vi "FPGA Server (9636).vi"() -> ()   [LabVIEW 2015]
doc: "This is the FPGA server for the sbRIO for the open-path cavity ring down."
uses:
  Rate.ctl
  <vilib>/Platform/TimedLoop/XDataNode/timing_clust.ctl
  <vilib>/Platform/TimedLoop/XDataNode/nitl_modes.ctl
  <vilib>/Platform/TimedLoop/XDataNode/wakeup.ctl
  <vilib>/rvi/FXPMathLib/FxpDiv/subVIs/nifxpmath_Div_SimConfig.ctl
  <vilib>/rvi/FXPMathLib/basic elements/FxpIntAccumulator/subVIs/nifxpmath_IntAccumulator_SimConfig.ctl
  <vilib>/rvi/Emulation/niFpgaGetClockAttributes.vi
  <vilib>/rvi/Emulation/niFpgaSctlEmulationGetInTimedLoop.vi
  <vilib>/rvi/Emulation/niFpgaEmulationReportErrorSimple.vi
  <vilib>/rvi/Emulation/niFpgaProcessEmulError.vi
  <vilib>/rvi/Memory/Memory_Emulation/nirvimemoryFastEmulation.vi
  <vilib>/rvi/Memory/Memory_Emulation/nirvimemoryEmulation.vi
  <vilib>/rvi/Emulation/niFpgaEmulationIsFPGAContextNoSignature.vi
  <vilib>/rvi/DataTransferAndStorage/Container/Common/niFpgaContainerGetUniqueNameForEmu.vi
  <vilib>/rvi/errors/nirviReportUnexpectedCaseInternalError (U32).vi
  <vilib>/rvi/interface/RandomDataEmulation/niFpgaRandomDataHandleErrors.vi
  <vilib>/rvi/Emulation/niFpgaCriticalErrorInLSC.vi
  <vilib>/rvi/eio/common/nirviEmuTemplateMethod_errors.vi
  <vilib>/rvi/Analysis/common/codeGenErrors/XNode/niFpgaXNodeCodeGenErrorHandle.vi
  <vilib>/rvi/FXPMathLib/basic elements/FxpIntAccumulator/simVIs/DllFxpIntAccumulator_sub.vi
  <vilib>/rvi/FXPMathLib/FxpDiv/simVIs/DllFxpDivTemp_sub.vi
  <vilib>/rvi/DataTransferAndStorage/Container/XNode/niFpgaContainer.xnode
  <vilib>/rvi/interface/RandomDataEmulation/nirviRandomDataFpgaReadWriteTemplate.vi
  <vilib>/eio/EIONode/EIONode.xnode
  <vilib>/rvi/Analysis/measure/mean-var-std/XNode/niFpgaMean-Var-Std.xnode
  <vilib>/Platform/TimedLoop/XDataNode/XDataNode.xnode
  <vilib>/rvi/FXPMathLib/basic elements/FxpIntAccumulator/XNode/nifxpmath_IntAccumulator.xnode
  <vilib>/rvi/FXPMathLib/FxpMul/XNode/nifxpmath_Multiplier.xnode
  <vilib>/rvi/FXPMathLib/FxpSub/XNode/nifxpmath_Sub.xnode
  <vilib>/rvi/FXPMathLib/FxpDiv/XNode/nifxpmath_Div.xnode
  <vilib>/Platform/TimedLoop/XDataNode/XDNodeRunTimeDep.lvlib
  <vilib>/rvi/FXPMathLib/sim/FxpSim.dll
panel:
  out "Rotronic":cluster{"RH":fxp<+,16,8>, "T":fxp<+/-,16,8>}
  out "CollectData":bool
  in  "max":i32
  in  "InvertLaser?":bool
  in  "LaserOff (us)":u32
  in  "Fans":T1
  in  "Reverse?":bool
  out "ShipError":bool
  out "EncodeLoop":bool
  out "ServoLoop":bool
  out "LaserLoop":bool
  out "HKLoop":bool
  out "ShipLoop":bool
  out "DataLoop":bool
  out "LF Data":T2
  in  "Low":u32 caption="Count(uSec)"
  in  "High":u32 caption="Count(uSec)"
  out "Delay Ticks":u32
  in  "Delay (us)":u16
  out "RequestLaser":bool
  out "Sample Ticks":u32
  in  "Pause Digitizer":bool
  in  "Sample Time (us)":u16
  in  "Rate":T3=3 items=["1 MHz"=20, "2 MHz"=10, "2.5 MHz"=8, "5 MHz"=4, "10 MHz"=2, "20MHz"=1]
  out "LaserOFF?":bool
  in  "Cylce (ticks)":u32=40000
  out "DataRead":bool
  out "dataready":bool
  out "NewData":u16
  out "NumElements":u32
  in  "Stop":bool
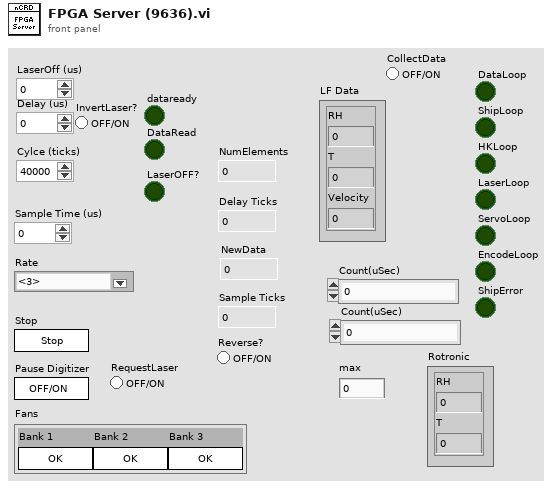
[diagram p1: front panel]
types:
  T1 = cluster{"Bank 1":bool, "Bank 2":bool, "Bank 3":bool}
  T2 = cluster{"RH":fxp<+,16,8>, "T":fxp<+/-,16,8>, "Velocity":fxp<+/-,16,8>}
  T3 = typedef "Rate.ctl" = u8
  T4 = typedef "XDNodeRunTimeDep.lvlib/timing_clust.ctl" = cluster{"Expected End [f-1]":u64, "Actual End [f-1]":u64, "Finished Late? [f-1]":bool, "Expected End [i-1]":u64, "Actual End [i-1]":u64, "Finished Late? [i-1]":bool, "Expected Start [i]":u64, "Actual Start [i]":u64, "Expected Start [f]":u64, "Actual Start [f]":u64, "Source Name":string, "Structure Name":string, "Period":i64, "Deadline":i64, "Offset":i64, "Start":i64, "Priority":i32, "Timeout":i32, "Mode":T5, "Wakeup Reason":T6, "Error":errorcluster, "Source Type":string, "Secondary Source Type":string, "Global End Time":u64, "Global Start Time":u64, "Frame Duration":u64, "Iteration Duration":u64, "Assigned CPU":i32, "I/O Scan Engine Mode":u32}
  T5 = typedef "XDNodeRunTimeDep.lvlib/nitl_modes.ctl" = enum32{"No Change", "Process missed periods, maintain original phase", "Discard missed periods, maintain original phase", "Process missed periods, ignore original phase", "Discard missed periods, ignore original phase"}
  T6 = typedef "XDNodeRunTimeDep.lvlib/wakeup.ctl" = enum32{"Normal", "Aborted", "Asynchronous wakeup", "Timing source error", "Timed loop error", "Timeout"}
  T7 = cluster{"fixed-point type":fxp<+/-,64,64>, "x+y":fxp<+/-,64,64>, "x+y":fxp<+/-,64,64>, "x+y":fxp<+/-,64,64>, "x+y":fxp<+/-,64,64>, "x+y":fxp<+/-,64,64>, "x+y":fxp<+/-,64,64>}
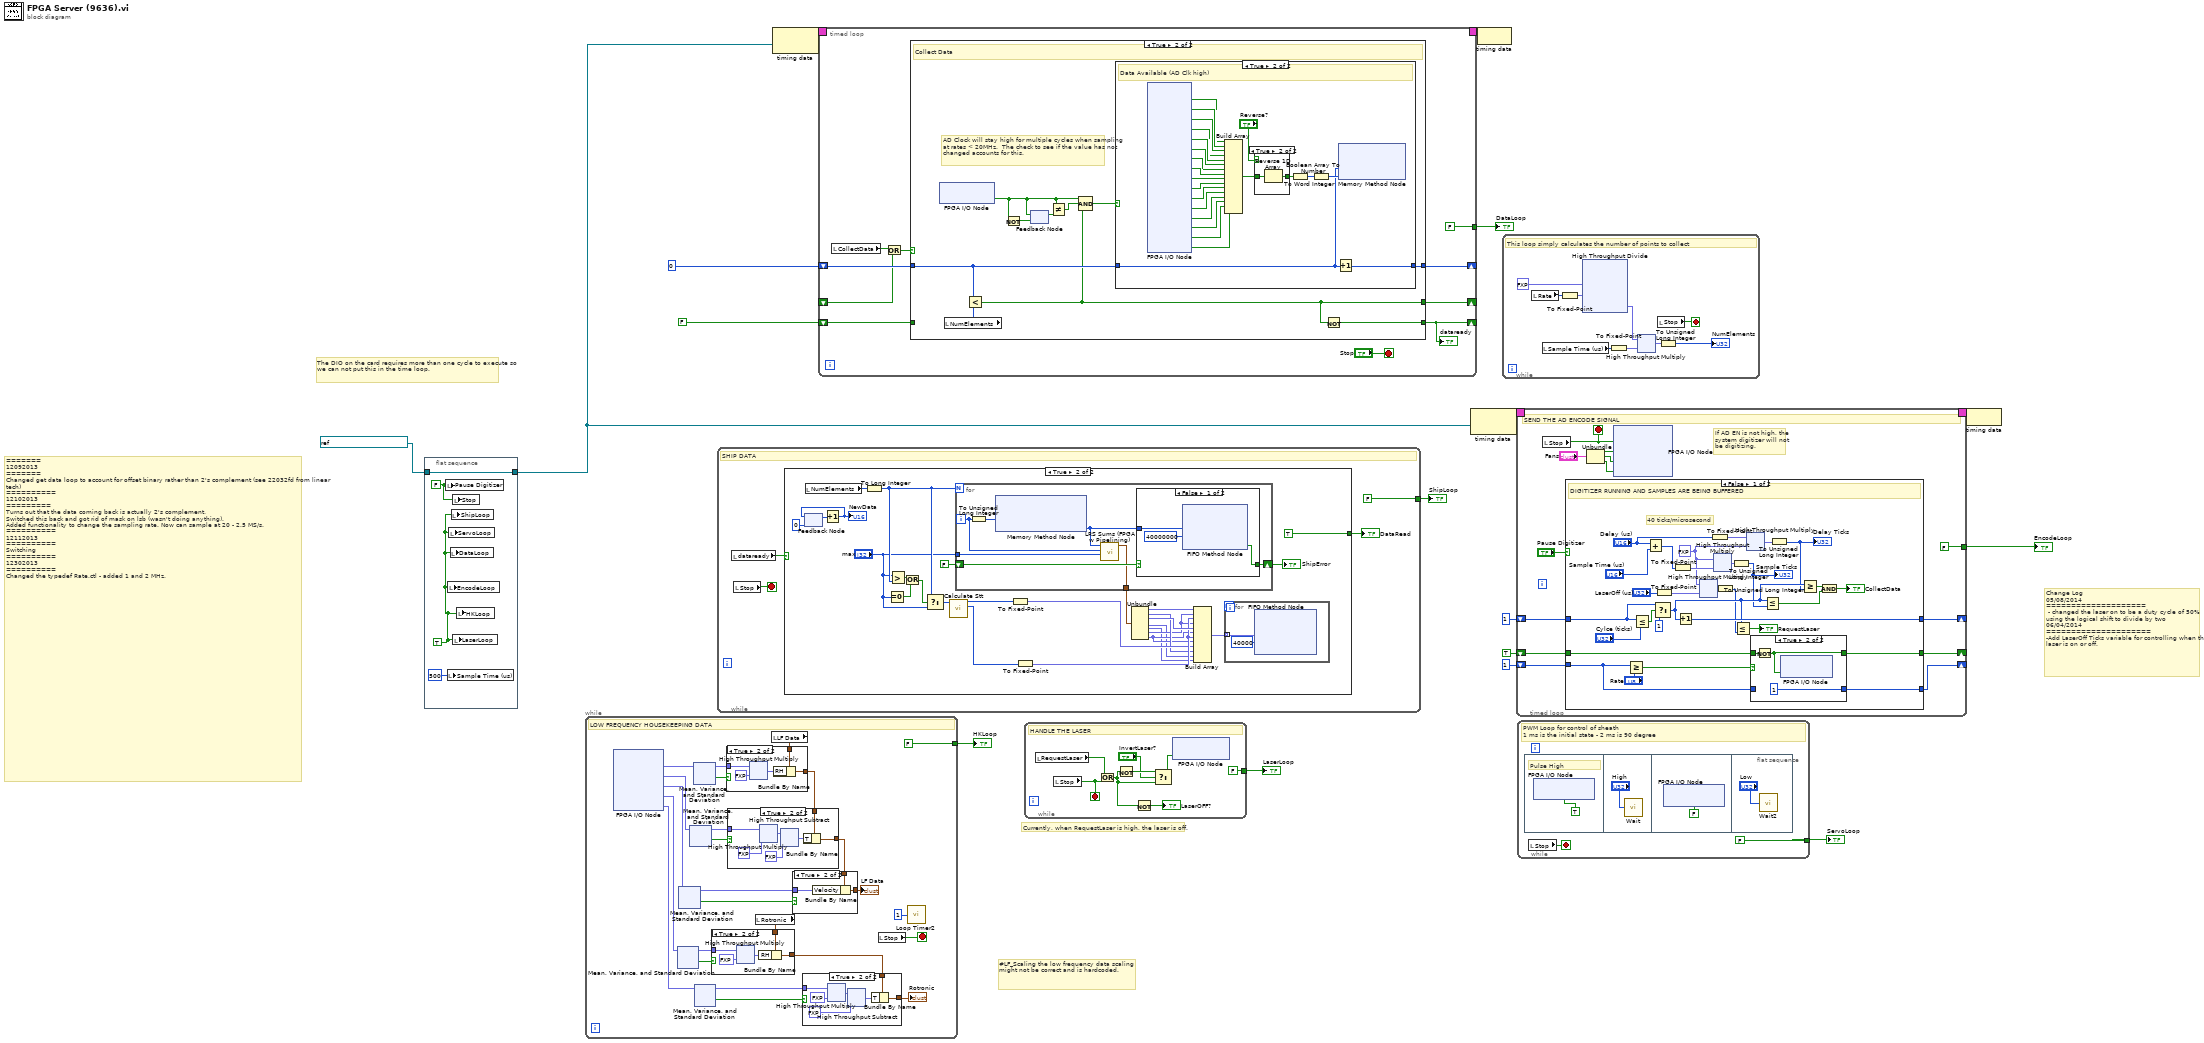
[diagram p0: block diagram]
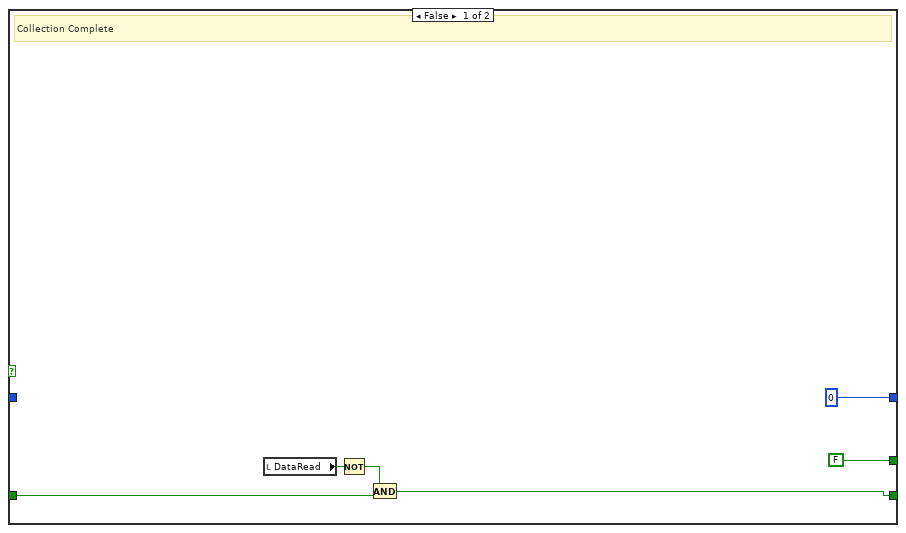
[diagram p2: hidden frame]
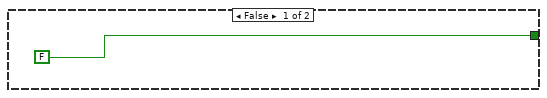
[diagram p10: hidden frame]
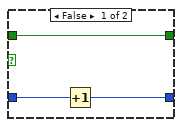
[diagram p12: hidden frame]
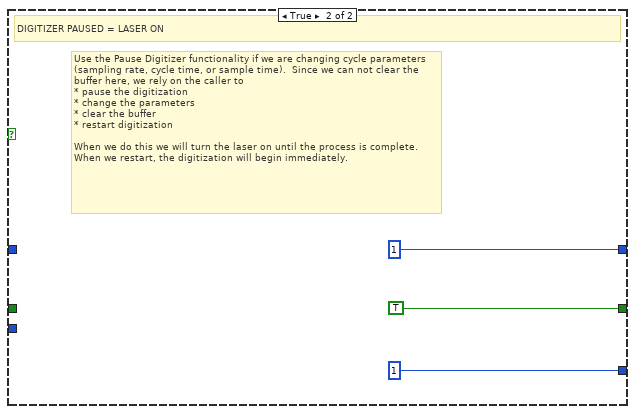
[diagram p13: hidden frame]
diagram:
  # "Change Log\n05/08/2014 \n====================\n - changed the laser on to be a duty cycle of 50% using the logical shift to divide by two\n06/04/2014\n=====================\n-Add LaserOff Ticks variable for controlling when the laser is on or off."
  # "Currently, when RequestLaser is high, the laser is off."
  # "#LF_Scaling the low frequency data scaling might not be correct and is hardcoded."
  # "The DIO on the card requires more than one cycle to execute so we can not put this in the time loop."
  # "=======\n12092013 \n=======\nChanged get data loop to account for offset binary rather than 2's complement (see 22032fd from linear tech)\n==========\n12102013\n=========\nTurns out that the data coming back is actually 2's complement. \nSwitched this back and got rid of mask on lsb (wasn't doing anything).\nAdded functionality to change the sampling rate. Now can sample at 20 - 2.5 MS/s.\n==========\n12112013\n==========\nSwitching\n==========\n12302013\n==========\nChanged the typedef Rate.ctl - added 1 and 2 MHz."
  n1 = flat-sequence {
    tunnel: refnum<k21> "40 MHz Onboard Clock" ("Source Name") -> [w21]
    tunnel: [w21] -> w1
    frame #0 {
      w19 = TRUE
      w20 = FALSE ("Pause Digitizer")
      n2 = local write "Pause Digitizer"(w20) -> ()
      n3 = local write "Sample Time (us)"(u16 500 ("Sample Time (us)")) -> ()
      n4 = local write "EncodeLoop"(w19) -> ()
      n5 = local write "ServoLoop"(w19) -> ()
      n6 = local write "DataLoop"(w19) -> ()
      n7 = local write "ShipLoop"(w19) -> ()
      n8 = local write "Stop"(w20) -> ()
      n9 = local write "LaserLoop"(w19) -> ()
      n10 = local write "HKLoop"(w19) -> ()
    }
  }
  n11 = while {
    tunnel: [FALSE] -> w10
    stop <- w32 stop-if-true
    # "LOW FREQUENCY HOUSEKEEPING DATA"
    n12 = xnode "FPGA I/O Node"() -> ("RH"=w45:fxp<+/-,24,5>, "TRH"=w44:fxp<+/-,24,5>, "uair"=w37:fxp<+/-,24,5>, "rot_RH"=w30:fxp<+/-,24,5>, "rot_TRH"=w27:fxp<+/-,24,5>)  [unwired: 5 in, 5 out]
    n13 = xnode "Mean, Variance, and Standard Deviation"("input data"=w30) -> ("mean"=w28:fxp<+/-,24,5>, "output valid"=w29:bool)  [unwired: 1 in]
    n14 = xnode "Mean, Variance, and Standard Deviation"("input data"=w37) -> ("mean"=w35:fxp<+/-,24,5>, "output valid"=w36:bool)  [unwired: 1 in]
    n15 = xnode "Mean, Variance, and Standard Deviation"("input data"=w44) -> ("mean"=w39:fxp<+/-,24,5>, "output valid"=w40:bool)  [unwired: 1 in]
    n16 = xnode "Mean, Variance, and Standard Deviation"("input data"=w45) -> ("mean"=w42:fxp<+/-,24,5>, "output valid"=w41:bool)  [unwired: 1 in]
    n17 = xnode "Mean, Variance, and Standard Deviation"("input data"=w27) -> ("mean"=w25:fxp<+/-,24,5>, "output valid"=w23:bool)  [unwired: 1 in]
    n18 = local read "Rotronic"() -> (w26:cluster{"RH":fxp<+,16,8>, "T":fxp<+/-,16,8>})
    n19 = case shown="True" w29 {
      tunnel: w28 -> [_ w60]
      tunnel: w26 -> [w55 w57]
      tunnel: [w55 w56] -> w24
      frame False {
      }
      frame True {
        n20 = xnode ("High Throughput Multiply")("x"=w60, "y"=fxp<+,8,8> 100.0) -> ("x*y"=w58:fxp<+/-,32,13>)
        n21 = Bundle By Name(cluster=w57, "RH"=w58) -> (w56:cluster{"RH":fxp<+,16,8>, "T":fxp<+/-,16,8>})
      }
    }
    n22 = local read "LF Data"() -> (w43:T2)
    n23 = case shown="True" w41 {
      tunnel: w43 -> [w301 w306]
      tunnel: w42 -> [_ w302]
      tunnel: [w301 w303] -> w38
      frame False {
      }
      frame True {
        n24 = xnode ("High Throughput Multiply")("x"=w302, "y"=fxp<+,8,8> 20.0) -> ("x*y"=w304:fxp<+/-,32,13>)
        n25 = Bundle By Name(cluster=w306, "RH"=w304) -> (w303:T2)
      }
    }
    n26 = case shown="True" w40 {
      tunnel: w38 -> [w293 w300]
      tunnel: w39 -> [_ w294]
      tunnel: [w293 w295] -> w34
      frame False {
      }
      frame True {
        n27 = xnode ("High Throughput Multiply")("x"=w294, "y"=fxp<+,8,8> 24.0) -> ("x*y"=w298:fxp<+/-,32,13>)
        n28 = xnode "High Throughput Subtract"("x"=w298, "y"=fxp<+/-,8,8> 40.0) -> ("x-y"=w296:fxp<+/-,33,14>)
        n29 = Bundle By Name(cluster=w300, "T"=w296) -> (w295:T2)
      }
    }
    n30 = case shown="True" w36 {
      tunnel: w34 -> [w289 w292]
      tunnel: w35 -> [_ w290]
      tunnel: [w289 w291] -> w33
      frame False {
      }
      frame True {
        n31 = Bundle By Name(cluster=w292, "Velocity"=w290) -> (w291:T2)
      }
    }
    "LF Data" <- w33
    n32 = case shown="True" w23 {
      tunnel: w25 -> [_ w54]
      tunnel: w24 -> [w47 w52]
      tunnel: [w47 w51] -> w22
      frame False {
      }
      frame True {
        n33 = xnode ("High Throughput Multiply")("x"=w54, "y"=fxp<+,8,8> 100.0) -> ("x*y"=w50:fxp<+/-,32,13>)
        n34 = xnode "High Throughput Subtract"("x"=w50, "y"=fxp<+/-,8,8> 40.0) -> ("x-y"=w48:fxp<+/-,33,14>)
        n35 = Bundle By Name(cluster=w52, "T"=w48) -> (w51:cluster{"RH":fxp<+,16,8>, "T":fxp<+/-,16,8>})
      }
    }
    "Rotronic" <- w22
    n36 = local read "Stop"() -> (w32:bool)
    n37 = call "Loop Timer2"("Count(mSec)"=u32 1 ("Count(Ticks)")) -> ()  [unwired: 1 out]
  }
  "HKLoop" <- w10
  n38 = while {
    tunnel: [FALSE] -> w11
    stop <- w462 stop-if-true
    # "SHIP DATA"
    n39 = local read "dataready"() -> (w461:bool)
    n40 = local read "Stop"() -> (w462:bool)
    n41 = case shown="True" w461 {
      tunnel: [FALSE TRUE] -> w460
      frame False {
      }
      frame True {
        n42 = feedback #1(u16 0) -> (w487:u16)
        n43 = local read "NumElements"() -> (w483:u32)
        n44 = Increment(x=w487) -> (x+1=w488:u16)
        "NewData" <- w488
        n45 = feedback-in #1(w488) -> ()
        n46 = To Long Integer(number=w483) -> (32bit integer=w468:i32)
        n47 = Equal To 0?(x="max") -> (x = 0?=w465:bool)
        n48 = Greater?(x="max", y=w468) -> (0:w466:bool)
        n49 = Or(x=w466, y=w465) -> (x .or. y?=w464:bool)
        n50 = Select(t=w468, s=w464, f="max") -> (s? t:f=w482:i32)
        n51 = call "Calculate Stt.vi"("N"=w482) -> ("St"=w480:i64, "Stt"=w481:i64)  [unwired: 9 in]
        n52 = for {
          N: w468 -> [_]
          shift-right: [w495] -> w485
          shift-left: FALSE ("Timed Out?") -> [w494]
          tunnel: [w490] -> w475
          tunnel: "max" -> [w491]
          i -> [w493]
          n53 = To Unsigned Long Integer(number=w493) -> (unsigned 32bit integer=w496:u32)
          n54 = xnode ("Memory Method Node")("Address"=w496) -> ("Data"=w492:i16)  [unwired: 1 in, 1 out]
          n55 = call "LRS Sums (FPGA w Pipelining).vi"("max"=w491, "i"=w493, "DataIn"=w492) -> ("DataOut"=w490:T7)  [unwired: 8 in]
          n56 = case shown="False" w494 {
            selector: w494 -> [_ w500]
            tunnel: w492 -> [w499 _]
            tunnel: [w498 w500] -> w495
            frame False {
              n57 = xnode ("FIFO Method Node")("Element"=w499, "Timeout"=40000000) -> ("Timed Out?"=w498:bool)  [unwired: 1 in, 1 out]
            }
            frame True {
            }
          }
        }
        "ShipError" <- w485
        n58 = To Fixed-Point(number=w481) -> (fixed-point=w476:fxp<+/-,64,64>)  [unwired: 1 in]
        n59 = To Fixed-Point(number=w480) -> (fixed-point=w477:fxp<+/-,64,64>)  [unwired: 1 in]
        n60 = Unbundle(w475) -> ("fixed-point type"=w479:fxp<+/-,64,64>, "x+y"=w474:fxp<+/-,64,64>, "x+y"=w478:fxp<+/-,64,64>, "x+y"=w471:fxp<+/-,64,64>, "x+y"=w470:fxp<+/-,64,64>, "x+y"=w473:fxp<+/-,64,64>, "x+y"=w472:fxp<+/-,64,64>)
        n61 = Build Array(w479, w473, w477, w473, w478, w472, w477, w472, w476, w474, w471, w470) -> (w469:fxp<+/-,64,64>[])
        n62 = for {
          tunnel: w469 -> [w502] mode=indexing
          n63 = xnode ("FIFO Method Node")("Element"=w502, "Timeout"=40000) -> ()  [unwired: 1 in, 2 out]
        }
      }
    }
    "DataRead" <- w460
  }
  "ShipLoop" <- w11
  n64 = node-c288(w1) -> (w6:T4)
  n65 = timed-loop {
    timing: w6 -> [_]
    timing-out: [_] -> w5
    shift-right: [w510] -> _
    shift-left: u32 0 -> [w509]
    shift-right: [w508] -> _
    shift-left: _ -> [w507]
    shift-right: [w505] -> _
    shift-left: FALSE -> [w504]
    tunnel: [FALSE] -> w2
    stop <- "Stop" stop-if-true
    n66 = local read "CollectData"() -> (w512:bool)
    n67 = Or(x=w512, y=w507) -> (x .or. y?=w511:bool)
    n68 = case shown="True" w511 {
      tunnel: [u32 0 w524] -> w510
      tunnel: w509 -> [_ w525]
      tunnel: [FALSE w520] -> w508
      tunnel: [w513 w519] -> w505
      tunnel: w504 -> [w514 _]
      frame False {
        # "Collection Complete"
        n69 = local read "DataRead"() -> (w516:bool)
        n70 = Not(x=w516) -> (.not. x?=w515:bool)
        n71 = And(x=w515, y=w514) -> (x .and. y?=w513:bool)
      }
      frame True {
        # "AD Clock will stay high for multiple cycles when sampling at rates < 20MHz.  The check to see if the value has not changed accounts for this."
        # "Collect Data"
        n72 = xnode "FPGA I/O Node"() -> ("AD CLK +"=w522:bool)  [unwired: 1 in, 1 out]
        n73 = local read "NumElements"() -> (w528:u32)
        n74 = Less?(x=w525, y=w528) -> (x < y?=w520:bool)
        n75 = Not(x=w522) -> (.not. x?=w526:bool)
        n76 = feedback #2(w526) -> (w527:bool)
        n77 = feedback-in #2(w522) -> ()
        n78 = Not Equal?(x=w522, y=w527) -> (x != y?=w523:bool)
        n79 = Compound Arithmetic op=AND(w522, w523, w520) -> (w521:bool)
        n80 = case shown="True" w521 {
          tunnel: w525 -> [w529 w531]
          tunnel: [w529 w532] -> w524
          frame False {
            # "Waiting (Clk previously high or currently low)"
          }
          frame True {
            # "Data Available (AD Clk high)"
            n81 = xnode "FPGA I/O Node"() -> ("AD0"=w533:bool, "AD1"=w534:bool, "AD2"=w535:bool, "AD3"=w536:bool, "AD4"=w537:bool, "AD5"=w538:bool, "AD6"=w539:bool, "AD7"=w540:bool, "AD8"=w541:bool, "AD9"=w542:bool, "AD10"=w543:bool, "AD11"=w544:bool, "AD12"=w545:bool, "AD13"=w546:bool, "AD14"=w547:bool, "AD15"=w548:bool)  [unwired: 16 in, 16 out]
            n82 = Build Array(w533, w534, w535, w536, w537, w538, w539, w540, w541, w542, w543, w544, w545, w546, w547, w548) -> (w551:bool[])
            n83 = case shown="True" "Reverse?" {
              tunnel: w551 -> [w553 w555]
              tunnel: [w553 w554] -> w552
              frame False {
              }
              frame True {
                n84 = Reverse 1D Array(array=w555) -> (reversed array=w554:bool[])
              }
            }
            n85 = Boolean Array To Number(Boolean array=w552) -> (number=w549:u16)
            n86 = To Word Integer(number=w549) -> (16bit integer=w550:i16)
            n87 = Increment(x=w531) -> (x+1=w532:u32)
            n88 = xnode ("Memory Method Node")("Address"=w531, "Data"=w550) -> ()  [unwired: 1 in, 1 out]
          }
        }
        n89 = Not(x=w520) -> (.not. x?=w519:bool)
      }
    }
    "dataready" <- w505
  }
  "DataLoop" <- w2
  n90 = while {
    tunnel: [FALSE] -> w9
    stop <- w564 stop-if-true
    # "HANDLE THE LASER"
    n91 = local read "RequestLaser"() -> (w565:bool)
    n92 = local read "Stop"() -> (w564:bool)
    n93 = Or(x=w565, y=w564) -> (x .or. y?=w559:bool)
    n94 = Not(x=w559) -> (.not. x?=w561:bool)
    n95 = Not(x=w559) -> (.not. x?=→"LaserOFF?":bool)
    n96 = Select(t=w561, s="InvertLaser?", f=w559) -> (s? t:f=w560:bool)
    n97 = xnode "FPGA I/O Node"("Laser Mod"=w560) -> ()  [unwired: 1 in, 1 out]
  }
  "LaserLoop" <- w9
  n98 = node-c288(w1) -> (w17:T4)
  n99 = node-c288(w5) -> ()
  n100 = while {
    stop <- w574 stop-if-true
    # "This loop simply calculates the number of points to collect"
    n101 = local read "Rate"() -> (w570:T3)
    n102 = local read "Sample Time (us)"() -> (w573:u16)
    n103 = To Fixed-Point(number=w570) -> (fixed-point=w569:fxp<+,8,8>)  [unwired: 1 in]
    n104 = xnode "High Throughput Divide"("x"=fxp<+,8,8> 20.0 ("Sample Time (us) 2"), "y"=w569) -> ("x/y"=w568:fxp<+,16,8>)
    n105 = To Fixed-Point(number=w573) -> (fixed-point=w572:fxp<+,16,16>)  [unwired: 1 in]
    n106 = xnode ("High Throughput Multiply")("x"=w568, "y"=w572) -> ("x*y"=w567:fxp<+,32,32>)
    n107 = local read "Stop"() -> (w574:bool)
    n108 = To Unsigned Long Integer(number=w567) -> (unsigned 32bit integer=→"NumElements":u32)
  }
  n109 = timed-loop {
    shift-right: [w610] -> _
    shift-left: TRUE -> [w611]
    timing: w17 -> [_]
    timing-out: [_] -> w16
    shift-right: [w612] -> _
    shift-left: u32 1 -> [w613]
    shift-right: [w609] -> _
    shift-left: u8 1 -> [w608]
    tunnel: [FALSE] -> w7
    stop <- w614 stop-if-true
    # "If AD EN is not high, the system digitizer will not be digitizing."
    # "SEND THE AD ENCODE SIGNAL"
    n110 = local read "Stop"() -> (w614:bool)
    n111 = case shown="False" "Pause Digitizer" {
      tunnel: w613 -> [w627 _]
      tunnel: [w642 u32 1] -> w612
      tunnel: w611 -> [w639 _]
      tunnel: [w638 TRUE ("Element")] -> w610
      tunnel: [w637 u8 1] -> w609
      tunnel: w608 -> [w636 _]
      frame False {
        w623 = fxp<+,8,8> 40.0 ("Sample Time (us) 2")
        # "40 ticks/microsecond"
        # "DIGITIZER RUNNING AND SAMPLES ARE BEING BUFFERED"
        n112 = Greater Or Equal?(x=w636, y="Rate") -> (x >= y?=w640:bool)
        n113 = Less Or Equal?(x=w627, y="Cylce (ticks)") -> (x <= y?=w644:bool)
        n114 = Add(x="Delay (us)", y="Sample Time (us)") -> (x+y=w633:u16)
        n115 = Select(t=w627, s=w644, f=u32 1) -> (s? t:f=w625:u32)
        n116 = To Fixed-Point(number="LaserOff (us)") -> (fixed-point=w621:fxp<+,32,32>)  [unwired: 1 in]
        n117 = To Fixed-Point(number=w633) -> (fixed-point=w634:fxp<+,16,16>)  [unwired: 1 in]
        n118 = Increment(x=w625) -> (x+1=w642:u32)
        n119 = xnode ("High Throughput Multiply")("x"=w623, "y"=w621) -> ("x*y"=w620:fxp<+,32,32>)
        n120 = To Fixed-Point(number="Delay (us)") -> (fixed-point=w630:fxp<+,16,16>)  [unwired: 1 in]
        n121 = xnode ("High Throughput Multiply")("x"=w623, "y"=w634) -> ("x*y"=w635:fxp<+,32,32>)
        n122 = To Unsigned Long Integer(number=w620) -> (unsigned 32bit integer=w619:u32)
        n123 = To Unsigned Long Integer(number=w635) -> (unsigned 32bit integer=w615:u32)
        "Sample Ticks" <- w615
        n124 = Less Or Equal?(x=w625, y=w619) -> (x <= y?=→"RequestLaser":bool)
        n125 = xnode ("High Throughput Multiply")("x"=w630, "y"=w623) -> ("x*y"=w629:fxp<+,32,32>)
        n126 = case shown="True" w640 {
          tunnel: w639 -> [w647 w650]
          tunnel: [w647 w649] -> w638
          tunnel: [w645 u8 1] -> w637
          tunnel: w636 -> [w646 _]
          frame False {
            n127 = Increment(x=w646) -> (x+1=w645:u8)
          }
          frame True {
            n128 = Not(x=w650) -> (.not. x?=w649:bool)
            n129 = xnode "FPGA I/O Node"("ENCODE"=w649) -> ()  [unwired: 1 in, 1 out]
          }
        }
        n130 = Less Or Equal?(x=w625, y=w615) -> (x <= y?=w632:bool)
        n131 = To Unsigned Long Integer(number=w629) -> (unsigned 32bit integer=w616:u32)
        "Delay Ticks" <- w616
        n132 = Greater Or Equal?(x=w625, y=w616) -> (x >= y?=w628:bool)
        n133 = And(x=w628, y=w632) -> (x .and. y?=→"CollectData":bool)
      }
      frame True {
        # "Use the Pause Digitizer functionality if we are changing cycle parameters (sampling rate, cycle time, or sample time).  Since we can not clear the buffer here, we rely on the caller to \n* pause the digitization\n* change the parameters\n* clear the buffer\n* restart digitization\n\nWhen we do this we will turn the laser on until the process is complete. When we restart, the digitization will begin immediately."
        # "DIGITIZER PAUSED = LASER ON"
      }
    }
    n134 = Unbundle("Fans") -> ("Bank 1"=w604:bool, "Bank 2"=w603:bool, "Bank 3"=w602:bool)
    n135 = xnode "FPGA I/O Node"("AD EN"=w614, "Fan Bank 1"=w604, "Fan Bank 2"=w603, "Fan Bank 3"=w602) -> ()  [unwired: 4 in, 4 out]
  }
  "EncodeLoop" <- w7
  n136 = while {
    tunnel: [FALSE] -> w8
    stop <- w657 stop-if-true
    # "PWM Loop for control of sheath\n1 ms is the initial state - 2 ms is 90 degree"
    n137 = flat-sequence {
      frame #0 {
        # "Pulse High"
        n138 = xnode "FPGA I/O Node"("Servo PWM"=TRUE ("Mod4/DIO0")) -> ()  [unwired: 1 in, 1 out]
      }
      frame #1 {
        n139 = call "Wait"("Count(uSec)"="High") -> ()  [unwired: 1 out]
      }
      frame #2 {
        n140 = xnode "FPGA I/O Node"("Servo PWM"=FALSE ("Mod4/DIO0")) -> ()  [unwired: 1 in, 1 out]
      }
      frame #3 {
        n141 = call "Wait2"("Count(Ticks)"="Low") -> ()  [unwired: 1 out]
      }
    }
    n142 = local read "Stop"() -> (w657:bool)
  }
  "ServoLoop" <- w8
  n143 = node-c288(w16) -> ()
